vi "Go_to_Idle.vi"(8 "error in (no error)":errorcluster, 11 "SI_Idle in":refnum<class "SI_Idle.lvclass">) -> (0 "error out":errorcluster, 3 "State out":refnum<class "State Actor.lvclass">)   [LabVIEW 2025, in "Sensor_Iterface.lvlib" / "SI_Idle.lvclass"]
uses:
  SI_Idle.lvclass
  SI_Idle.lvclass/SI_Idle.ctl
  C:/Users/halstead_rideriver/Documents/Labview_Practice/ATM_Machine_Actor Framework/ATM_ACTORFW/Sensor_Iterface/Sensor_Iterface/Sensor_Iterface.lvclass
  C:/Program Files (x86)/National Instruments/LabVIEW 2025/vi.lib/ni/Actors/State Actor/State Actor/State Actor.lvclass
  C:/Program Files (x86)/National Instruments/LabVIEW 2025/vi.lib/ActorFramework/Actor/Actor.lvclass
  C:/Users/halstead_rideriver/Documents/Labview_Practice/ATM_Machine_Actor Framework/ATM_ACTORFW/Sensor_Iterface/SI_Idle/SI_Idle.lvclass
  <vilib>/ni/Actors/State Actor/State Actor/State Actor.lvclass
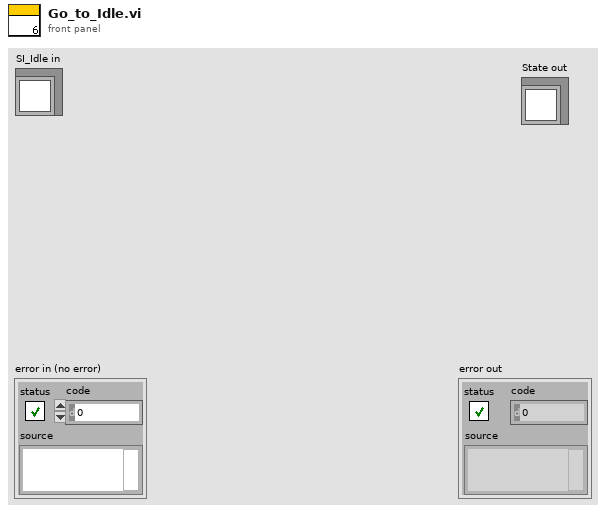
[diagram p1: front panel]
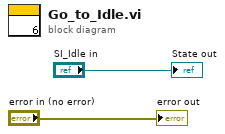
[diagram p0: block diagram]
diagram:
  "error out" <- "error in (no error)"
  "State out" <- "SI_Idle in"
